vi "Time_Converter.vi"(0 "InputSeconds":dbl) -> (4 "Hour":dbl, 6 "Minutes":dbl, 8 "Seconds":dbl, 10 "MilliSeconds":dbl)   [LabVIEW 2025]
doc: "This VI Converts Seconds into Hour, Minutes, Seconds, MilliSeconds"
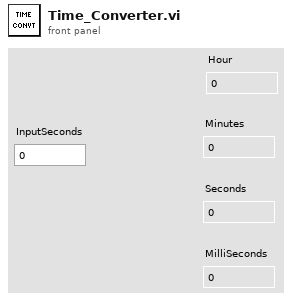
[diagram p1: front panel]
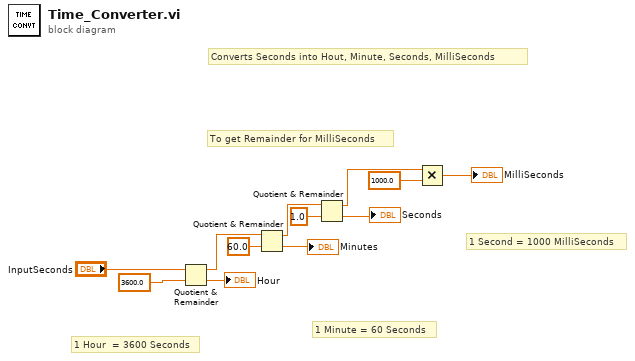
[diagram p0: block diagram]
diagram:
  # "1 Second = 1000 MilliSeconds"
  # "To get Remainder for MilliSeconds"
  # "1 Minute = 60 Seconds"
  # "1 Hour  = 3600 Seconds"
  # "Converts Seconds into Hout, Minute, Seconds, MilliSeconds"
  n1 = Quotient & Remainder(x="InputSeconds", y=3600.0) -> (x-y*floor(x/y)=w9:dbl, floor(x/y)=→"Hour":dbl)
  n2 = Quotient & Remainder(x=w9, y=60.0) -> (x-y*floor(x/y)=w6:dbl, floor(x/y)=→"Minutes":dbl)
  n3 = Quotient & Remainder(x=w6, y=1.0) -> (x-y*floor(x/y)=w3:dbl, floor(x/y)=→"Seconds":dbl)
  n4 = Multiply(x=w3, y=1000.0) -> (x*y=→"MilliSeconds":dbl)
